vi "Save Test Config.vi"(0 "Header Info":string[](array[string]), 1 "SNs":string[](array[string]), 2 "Profile":string[][](array[string]), 3 "VoltageLoc":string, 4 "CurrentLoc":string, 7 "Filepath":path, 11 "Error In":errorcluster) -> (15 "Error Out":errorcluster)   [LabVIEW 2013]
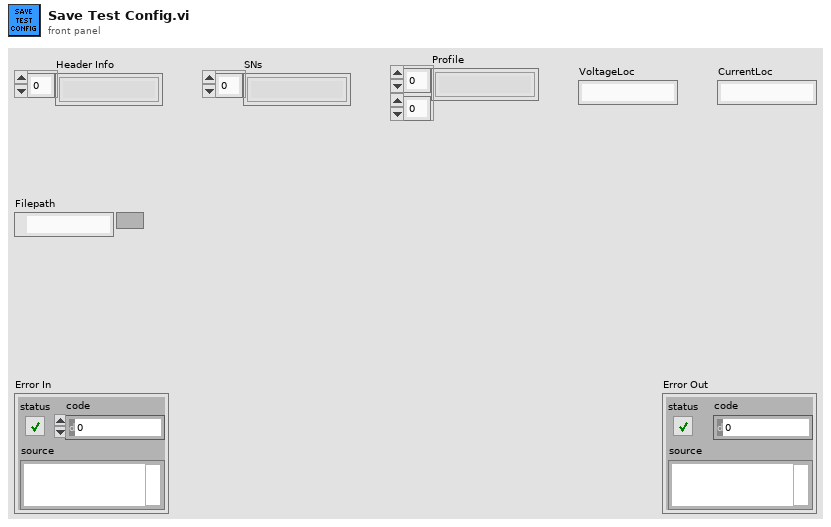
[diagram p1: front panel]
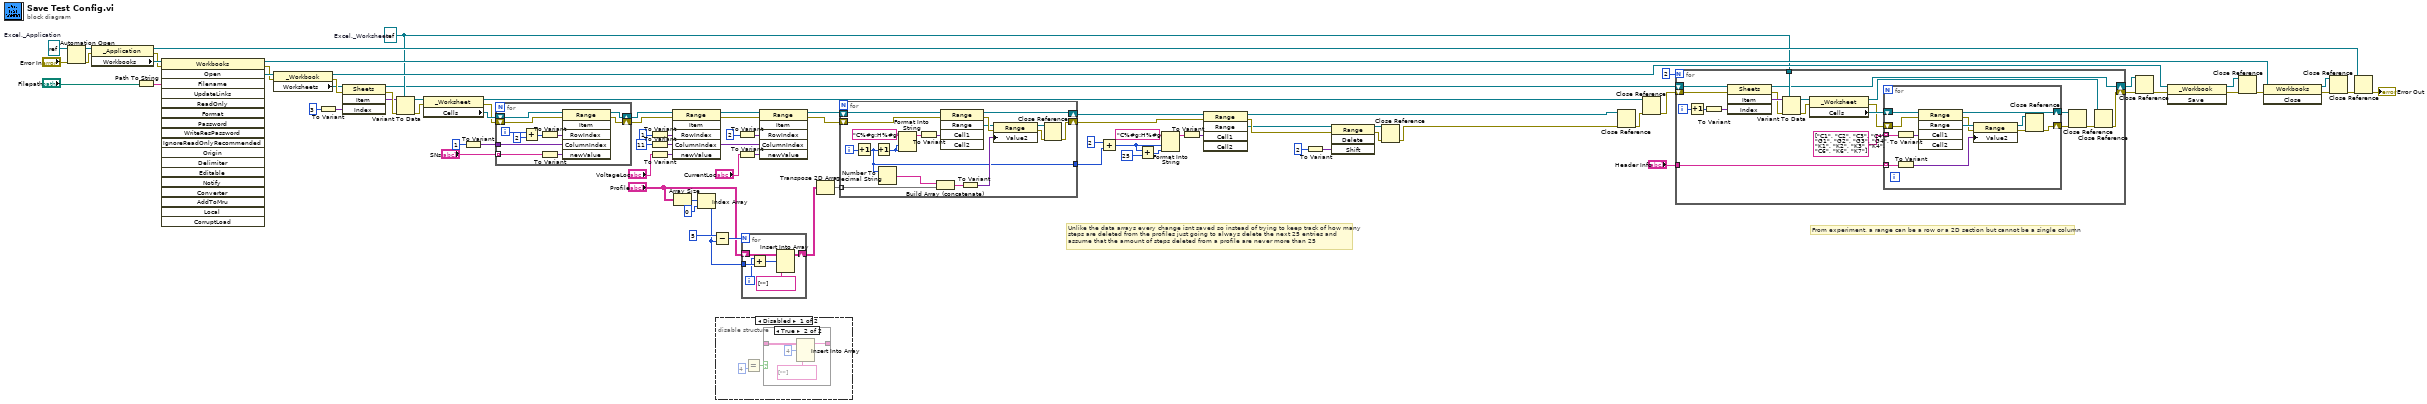
[diagram p0: block diagram]
diagram:
  w55 = refnum<k7> refnum  # Excel._Worksheet
  w82 = refnum<k7> refnum  # Excel._Application
  # "Unlike the data arrays every change isnt saved so instead of trying to keep track of how many\nsteps are deleted from the profiles just going to always delete the next 25 entries and\nassume that the amount of steps deleted from a profile are never more than 25"
  # "From experiment, a range can be a row or a 2D section but cannot be a single column"
  n1 = Automation Open(error in (no error)="Error In", Automation Refnum=w82) -> (Automation Refnum=w83:refnum<k7>, error out=w84:errorcluster)  [unwired: 2 in]
  n2 = property class="_Application"(reference=w83, error in=w84) -> (reference out=w75:refnum<k7>, error out=w76:errorcluster, "Workbooks"=w85:refnum<k7>)
  n3 = Path To String(path="Filepath") -> (string=w72:string)
  n4 = invoke class="Workbooks" method="Open"(reference=w85, error in=w76, "Filename"=w72) -> (reference out=w79:refnum<k7>, error out=w74:errorcluster, "Open"=w81:refnum<k7>)  [unwired: 15 in, 15 out]
  n5 = property class="_Workbook"(reference=w81, error in=w74) -> (reference out=w68:refnum<k7>, error out=w58:errorcluster, "Worksheets"=w57:refnum<k7>)
  n6 = To Variant(anything=3) -> (Variant=w59:variant)
  n7 = invoke class="Sheets" method="Item"(reference=w57, error in=w58, "Index"=w59) -> (reference out=w44:refnum<k7>, error out=w61:errorcluster, "Item"=w60:variant)  [unwired: 1 in, 1 out]
  n8 = Variant To Data(error in=w61, type=w55, Variant=w60) -> (data=w62:refnum<k7>, error out=w63:errorcluster)
  n9 = property class="_Worksheet"(reference=w62, error in=w63) -> (reference out=w43:refnum<k7>, error out=w34:errorcluster, "Cells"=w37:refnum<k7>)
  n10 = To Variant(anything=1 ("y")) -> (Variant=w35:variant)
  n11 = for {
    tunnel: "SNs" -> [w93] mode=indexing
    tunnel: w35 -> [w89]
    shift-right: [w87] -> w33
    shift-left: w37 -> [w94]
    shift-right: [w86] -> w32
    shift-left: w34 -> [w88]
    i -> [w91]
    n12 = Add(x=w91, y=2) -> (x+y=w90:i32)
    n13 = To Variant(anything=w90) -> (Variant=w96:variant)
    n14 = To Variant(anything=w93) -> (Variant=w95:variant)
    n15 = invoke class="Range" method="Item"(reference=w94, error in=w88, "RowIndex"=w96, "ColumnIndex"=w89, "newValue"=w95) -> (reference out=w87:refnum<k7>, error out=w86:errorcluster)  [unwired: 1 in, 4 out]
  }
  n16 = To Variant(anything=1) -> (Variant=w38:variant)
  n17 = To Variant(anything=11) -> (Variant=w39:variant)
  n18 = To Variant(anything="VoltageLoc") -> (Variant=w53:variant)
  n19 = invoke class="Range" method="Item"(reference=w33, error in=w32, "RowIndex"=w38, "ColumnIndex"=w39, "newValue"=w53) -> (reference out=w54:refnum<k7>, error out=w46:errorcluster)  [unwired: 1 in, 4 out]
  n20 = Array Size(array="Profile") -> (size(s)=w7:i32[])
  n21 = Index Array(array=w7, index=0) -> (element=w2:i32)
  n22 = Subtract(x=5 ("y"), y=w2) -> (x-y=w4:i32)
  n23 = disable-structure shown="Disabled" {
    frame Disabled {
      n24 = Equal?(y=4) -> (x = y?=w97:bool)  [unwired: 1 in]
      n25 = case shown="True" w97 {
        tunnel: _ -> [w99 w103]
        tunnel: [w99 w102] -> _
        frame False {
        }
        frame True {
          n26 = Insert Into Array(array=w103, index (row)=4, new element=string[] [""]) -> (w102:string[])  [unwired: 1 in]
        }
      }
    }
    frame Enabled {
    }
  }
  n27 = To Variant(anything=2) -> (Variant=w40:variant)
  n28 = To Variant(anything="CurrentLoc") -> (Variant=w52:variant)
  n29 = for {
    N: w4 -> [_]
    shift-right: [w107] -> w1
    shift-left: "Profile" -> [w108]
    tunnel: w2 -> [w105]
    i -> [w104]
    n30 = Add(x=w104, y=w105) -> (x+y=w106:i32)
    n31 = Insert Into Array(array=w108, index (row)=w106, new element=string[] [""]) -> (w107:string[][])  [unwired: 1 in]
  }
  n32 = invoke class="Range" method="Item"(reference=w54, error in=w46, "RowIndex"=w40, "ColumnIndex"=w39, "newValue"=w52) -> (reference out=w31:refnum<k7>, error out=w45:errorcluster)  [unwired: 1 in, 4 out]
  n33 = Transpose 2D Array(2D array=w1) -> (transposed array=w30:string[][])
  n34 = for {
    shift-right: [w126] -> w24
    shift-left: w31 -> [w118]
    shift-right: [w117] -> w25
    shift-left: w45 -> [w127]
    tunnel: w30 -> [w113] mode=indexing
    tunnel: [w111] -> w14
    i -> [w114]
    n35 = Increment(x=w114) -> (x+1=w111:i32)
    n36 = Increment(x=w111) -> (x+1=w115:i32)
    n37 = Number To Decimal String(number=w111) -> (decimal integer string=w110:string)  [unwired: 1 in]
    n38 = Format Into String(format string="C%#g:H%#g", w115, w115) -> (resulting string=w119:string)  [unwired: 2 in, 1 out]
    n39 = To Variant(anything=w119) -> (Variant=w125:variant)
    n40 = Build Array (concatenate)(w110, w113) -> (w112:string[])
    n41 = invoke class="Range" method="Range"(reference=w118, error in=w127, "Cell1"=w125) -> (reference out=w126:refnum<k7>, error out=w123:errorcluster, "Range"=w122:refnum<k7>)  [unwired: 2 in, 2 out]
    n42 = To Variant(anything=w112) -> (Variant=w124:variant)
    n43 = property class="Range"(reference=w122, error in=w123, "Value2"=w124) -> (reference out=w121:refnum<k7>, error out=w120:errorcluster)
    n44 = Close Reference(reference=w121, error in (no error)=w120) -> (error out=w117:errorcluster)
  }
  n45 = Add(x=2 ("y"), y=w14) -> (x+y=w13:i32)
  n46 = Add(x=w13, y=25) -> (x+y=w15:i32)
  n47 = Format Into String(format string="C%#g:H%#g", w13, w15) -> (resulting string=w18:string)  [unwired: 2 in, 1 out]
  n48 = To Variant(anything=w18) -> (Variant=w23:variant)
  n49 = invoke class="Range" method="Range"(reference=w24, error in=w25, "Cell1"=w23) -> (reference out=w9:refnum<k7>, error out=w22:errorcluster, "Range"=w21:refnum<k7>)  [unwired: 2 in, 2 out]
  n50 = To Variant(anything=2 ("y")) -> (Variant=w11:variant)
  n51 = invoke class="Range" method="Delete"(reference=w21, error in=w22, "Shift"=w11) -> (reference out=w20:refnum<k7>, error out=w19:errorcluster)  [unwired: 1 in, 2 out]
  n52 = Close Reference(reference=w20, error in (no error)=w19) -> (error out=w8:errorcluster)
  n53 = Close Reference(reference=w9, error in (no error)=w8) -> (error out=w42:errorcluster)
  n54 = Close Reference(reference=w43, error in (no error)=w42) -> (error out=w41:errorcluster)
  n55 = for {
    N: 2 -> [_]
    tunnel: w55 -> [w142]
    shift-right: [w133] -> w67
    shift-left: w41 -> [w143]
    shift-right: [w132] -> w66
    shift-left: w44 -> [w144]
    tunnel: "Header Info" -> [w129]
    i -> [w131]
    n56 = Increment(x=w131) -> (x+1=w130:i32)
    n57 = To Variant(anything=w130) -> (Variant=w147:variant)
    n58 = invoke class="Sheets" method="Item"(reference=w144, error in=w143, "Index"=w147) -> (reference out=w132:refnum<k7>, error out=w145:errorcluster, "Item"=w146:variant)  [unwired: 1 in, 1 out]
    n59 = Variant To Data(error in=w145, type=w142, Variant=w146) -> (data=w141:refnum<k7>, error out=w140:errorcluster)
    n60 = property class="_Worksheet"(reference=w141, error in=w140) -> (reference out=w138:refnum<k7>, error out=w134:errorcluster, "Cells"=w135:refnum<k7>)
    n61 = for {
      shift-right: [w154] -> w136
      shift-left: w134 -> [w159]
      shift-right: [w153] -> w137
      shift-left: w135 -> [w152]
      tunnel: w129 -> [w151] mode=indexing
      tunnel: string[] ["C1", "C2", "C3", "C4", "G1", "G2", "G3", "G4", "K1", "K2", "K3", "K4", "C6", "K6", "K7"] -> [w150] mode=indexing
      n62 = To Variant(anything=w150) -> (Variant=w157:variant)
      n63 = To Variant(anything=w151) -> (Variant=w155:variant)
      n64 = invoke class="Range" method="Range"(reference=w152, error in=w159, "Cell1"=w157) -> (reference out=w153:refnum<k7>, error out=w156:errorcluster, "Range"=w158:refnum<k7>)  [unwired: 2 in, 2 out]
      n65 = property class="Range"(reference=w158, error in=w156, "Value2"=w155) -> (reference out=w149:refnum<k7>, error out=w148:errorcluster)
      n66 = Close Reference(reference=w149, error in (no error)=w148) -> (error out=w154:errorcluster)
    }
    n67 = Close Reference(reference=w137, error in (no error)=w136) -> (error out=w139:errorcluster)
    n68 = Close Reference(reference=w138, error in (no error)=w139) -> (error out=w133:errorcluster)
  }
  n69 = Close Reference(reference=w66, error in (no error)=w67) -> (error out=w73:errorcluster)
  n70 = invoke class="_Workbook" method="Save"(reference=w68, error in=w73) -> (reference out=w69:refnum<k7>, error out=w70:errorcluster)  [unwired: 1 in, 1 out]
  n71 = Close Reference(reference=w69, error in (no error)=w70) -> (error out=w71:errorcluster)
  n72 = invoke class="Workbooks" method="Close"(reference=w79, error in=w71) -> (reference out=w78:refnum<k7>, error out=w77:errorcluster)  [unwired: 1 in, 1 out]
  n73 = Close Reference(reference=w78, error in (no error)=w77) -> (error out=w80:errorcluster)
  n74 = Close Reference(reference=w75, error in (no error)=w80) -> (error out=→"Error Out":errorcluster)
